vi "RegisterSubPub.vi"(1 "Parameters":string[](array[string]), 2 "MethodName":string) -> (0 "XML":string)   [LabVIEW 2012]
doc: "Builds XML for registerPublisher and registerSubscriber calls.\nParams are\n - callerid\n - topic\n - type\n - uri\nMethodName is registerPublisher or registerSubscriber"
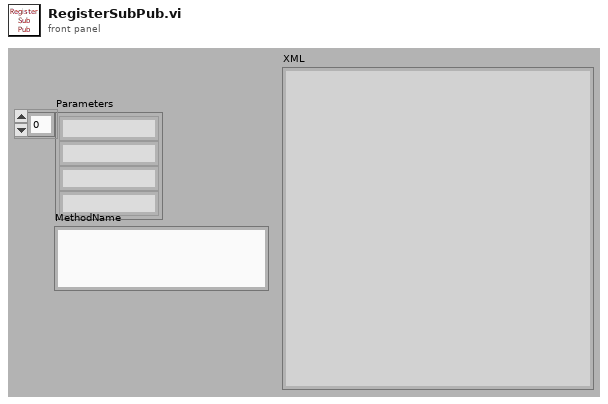
[diagram p1: front panel]
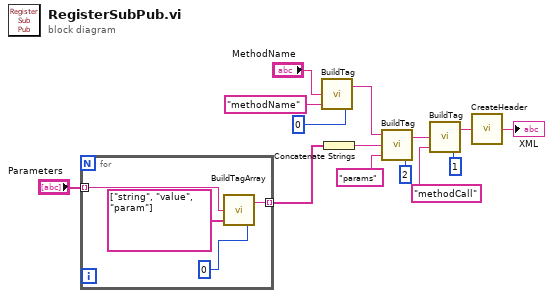
[diagram p0: block diagram]
diagram:
  n1 = for {
    tunnel: "Parameters" -> [w18] mode=indexing
    tunnel: [w16] -> w13 mode=indexing
    n2 = call "BuildTagArray.vi"("Indent"=i8 0, "tags"=string[] ["string", "value", "param"], "value"=w18) -> ("string out"=w16:string)  [unwired: 1 in]
  }
  n3 = call "BuildTag.vi"("Indent"=i8 0, "tag"="methodName", "value"="MethodName") -> ("string out"=w10:string)  [unwired: 1 in]
  n4 = Concatenate Strings(w13) -> (w8:string)
  n5 = call "BuildTag.vi"("Indent"=i8 2, "tag"="params", "value"=w8, "string in"=w10) -> ("string out"=w5:string)
  n6 = call "BuildTag.vi"("Indent"=i8 1, "tag"="methodCall", "value"=w5) -> ("string out"=w2:string)  [unwired: 1 in]
  n7 = call "CreateHeader.vi"("Content"=w2) -> ("XML"=→"XML":string)
